vi "UI_Status.vi"(7 "write?":bool, 8 "error in (no error)":errorcluster caption="错误输入（无错误）", 10 "menu status in":T1={"type"=2, "scantime"=30, "highspd"=FALSE, "disp"=TRUE, "save"=FALSE, "hl"=FALSE, "ID合并"=FALSE, "Rfun"=2, "Tfun"=2, "chk1"=FALSE, "chk2"=FALSE, "format"=enum."hex", "rateR1"=TRUE, "rateR2"=TRUE, "rateT1"=TRUE, "rateT2"=TRUE, "RcvE1"=TRUE, "RcvE2"=TRUE, "TSFormat"=enum."原始值", "RcvLen"=48}, 11 "VI ref":refnum<vi>) -> (0 "error out":errorcluster caption="错误输出", 3 "menu status in out":T1={"type"=2, "scantime"=30, "highspd"=FALSE, "disp"=TRUE, "save"=FALSE, "hl"=FALSE, "ID合并"=FALSE, "Rfun"=2, "Tfun"=2, "chk1"=FALSE, "chk2"=FALSE, "format"=enum."hex", "rateR1"=TRUE, "rateR2"=TRUE, "rateT1"=TRUE, "rateT2"=TRUE, "RcvE1"=TRUE, "RcvE2"=TRUE, "TSFormat"=enum."原始值", "RcvLen"=48})   [LabVIEW 2011]
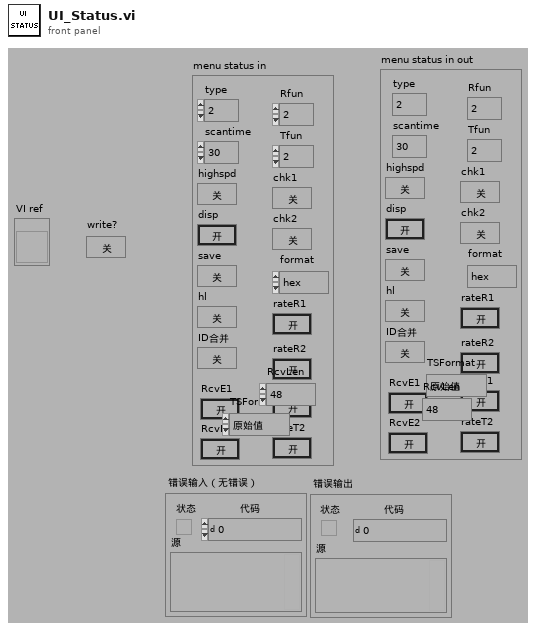
[diagram p1: front panel]
types:
  T1 = cluster{"type":u16, "scantime":u16, "highspd":bool, "disp":bool, "save":bool, "hl":bool, "ID合并":bool, "Rfun":u16, "Tfun":u16, "chk1":bool, "chk2":bool, "format":enum16{"hex", "dec", "oct", "bin"}, "rateR1":bool, "rateR2":bool, "rateT1":bool, "rateT2":bool, "RcvE1":bool, "RcvE2":bool, "TSFormat":enum16{"原始值", "实际值"}, "RcvLen":i16}
  T2 = cluster{"类ID":u32, "标签.文本":string, "禁用":enum8{"Enabled", "Disabled", "Disabled and Grayed Out"}, "可见":bool, "值":variant}[]
  T3 = cluster{"类ID":u32, "标签.文本":string, "禁用":enum8{"Enabled", "Disabled", "Disabled and Grayed Out"}, "可见":bool, "值":variant}
  T4 = enum8{"Enabled", "Disabled", "Disabled and Grayed Out"}
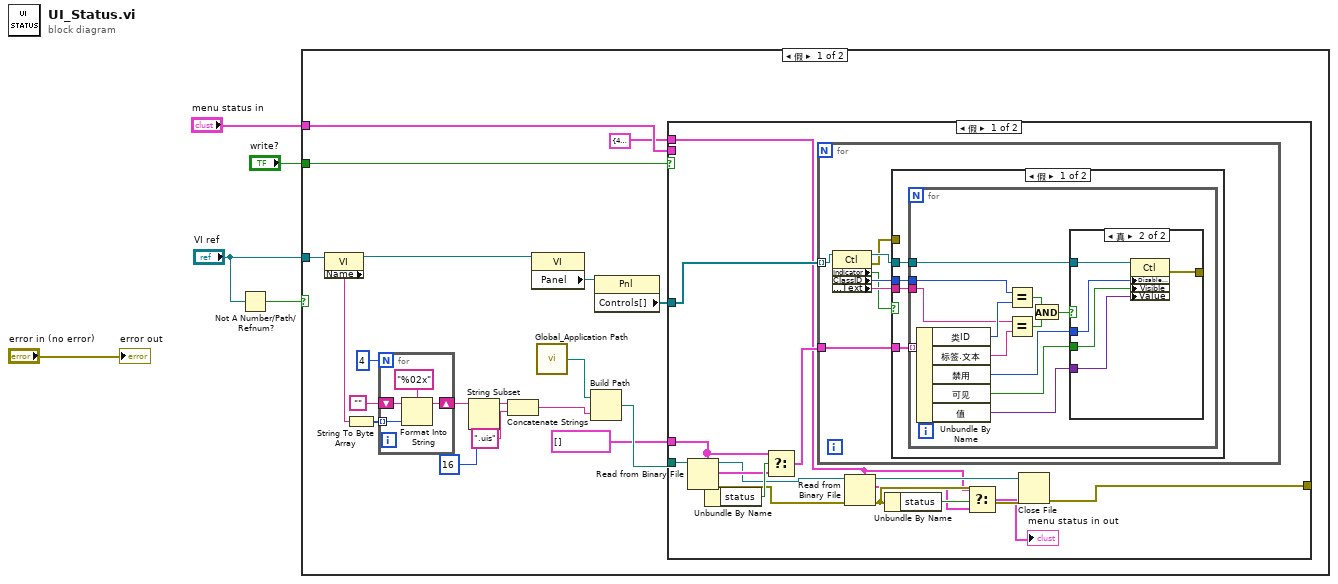
[diagram p0: block diagram]
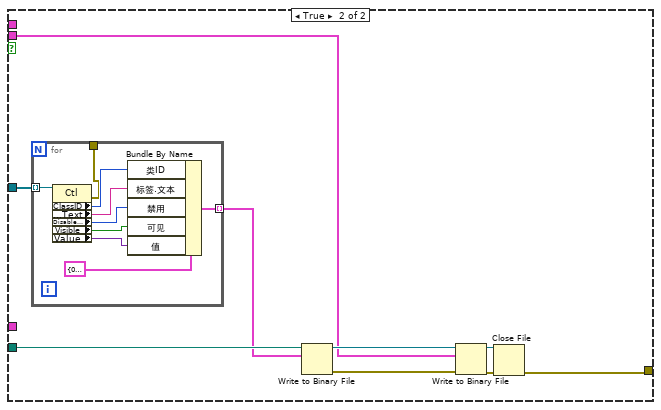
[diagram p4: hidden frame]
diagram:
  n1 = Not A Number/Path/Refnum?(number/path/refnum="VI ref") -> (NaN/Path/Refnum?=w1:bool)
  n2 = case shown="假" w1 {
    tunnel: "VI ref" -> [w24 _]
    tunnel: "write?" -> [w20 _]
    tunnel: "menu status in" -> [w17 _]
    frame False {
      n3 = property class="VI"(reference=w24) -> (reference out=w23:refnum<vi>, "Name"=w14:string)  [unwired: 1 in, 1 out]
      n4 = String To Byte Array(string=w14) -> (unsigned byte array=w15:u8[])
      n5 = for {
        N: 4 -> [_]
        tunnel: w15 -> [w28] mode=indexing
        shift-right: [w25] -> w13
        shift-left: "" -> [w26]
        n6 = Format Into String(format string="%02x" ("格式字符串"), initial string=w26, w28) -> (resulting string=w25:string)  [unwired: 1 in, 1 out]
      }
      n7 = String Subset(string=w13, length (rest)=16 ("长度（剩余）")) -> (substring=w10:string)  [unwired: 1 in]
      n8 = Concatenate Strings(w10, ".uis" ("字符串")) -> (w11:string)
      n9 = property class="VI"(reference=w23) -> ("Panel"=w22:refnum<vi>)  [unwired: 1 in, 2 out]
      n10 = call "Global_Application Path.vi"() -> ("程序路径"=w8:path)  [unwired: 1 in]
      n11 = Build Path(base path=w8, name or relative path=w11) -> (appended path=w19:path)
      n12 = property class="Pnl"(reference=w22) -> ("Controls[]"=w21:refnum<vi>[])  [unwired: 1 in, 2 out]
      n13 = case shown="假" w20 {
        tunnel: w21 -> [w37 w80]
        tunnel: w19 -> [w43 w79]
        tunnel: T2 [] -> [w41 _]
        tunnel: [w39 w77] -> _
        tunnel: T1 {"type"=4, "scantime"=30, "highspd"=FALSE, "disp"=TRUE, "save"=FALSE, "hl"=FALSE, "ID合并"=FALSE, "Rfun"=2, "Tfun"=2, "chk1"=FALSE, "chk2"=FALSE, "format"=enum."hex", "rateR1"=TRUE, "rateR2"=TRUE, "rateT1"=TRUE, "rateT2"=TRUE, "RcvE1"=TRUE, "RcvE2"=TRUE, "TSFormat"=enum."原始值", "RcvLen"=2500} ("menu status in out") -> [w31 _]
        tunnel: w17 -> [_ w72]
        frame False {
          n14 = Read from Binary File(5:w41, 11:w43) -> (0:w34:errorcluster, 2:w40:T2, 3:w36:refnum<file>)  [unwired: 4 in, 1 out]
          n15 = Unbundle By Name(w34) -> ("status"=w42:bool)
          n16 = Select(t=w41, s=w42, f=w40) -> (s? t:f=w38:T2)
          n17 = for {
            tunnel: w38 -> [w49]
            tunnel: w37 -> [w50] mode=indexing
            n18 = property class="Ctl"(reference=w50) -> (reference out=w48:refnum<vi>, error out=w44:errorcluster, "Indicator"=w45:bool, "ClassID"=w47:u32, "Label.Text"=w46:string)  [unwired: 1 in]
            n19 = case shown="假" w45 {
              tunnel: w49 -> [w54 _]
              tunnel: w48 -> [w53 _]
              tunnel: w47 -> [w52 _]
              tunnel: w46 -> [w51 _]
              tunnel: w44 -> [_ _]
              frame False {
                n20 = for {
                  tunnel: w54 -> [w66] mode=indexing
                  tunnel: w53 -> [w58]
                  tunnel: w52 -> [w65]
                  tunnel: w51 -> [w63]
                  n21 = Unbundle By Name(w66) -> ("类ID"=w64:u32, "标签.文本"=w62:string, "禁用"=w57:T4, "可见"=w56:bool, "值"=w55:variant)
                  n22 = Equal?(x=w65, y=w64) -> (x = y?=w61:bool)
                  n23 = Equal?(x=w63, y=w62) -> (x = y?=w60:bool)
                  n24 = And(x=w61, y=w60) -> (x .and. y?=w59:bool)
                  n25 = case shown="真" w59 {
                    tunnel: w58 -> [_ w71]
                    tunnel: w57 -> [_ w70]
                    tunnel: w56 -> [_ w69]
                    tunnel: w55 -> [_ w68]
                    tunnel: [_ w67] -> _
                    frame False {
                    }
                    frame True {
                      n26 = property class="Ctl"(reference=w71, "DisabledEnum"=w70, "Visible"=w69, "Value"=w68) -> (error out=w67:errorcluster)  [unwired: 1 in, 1 out]
                    }
                  }
                }
              }
              frame True {
              }
            }
          }
          n27 = Read from Binary File(5:w31, 8:w34, 11:w36) -> (0:w33:errorcluster, 2:w30:T1, 3:w35:refnum<file>)  [unwired: 3 in, 1 out]
          n28 = Unbundle By Name(w33) -> ("status"=w32:bool)
          n29 = Select(t=w31, s=w32, f=w30) -> (s? t:f=→"menu status in out":T1)
          n30 = Close File(refnum=w35, error in=w33) -> (error out=w39:errorcluster)  [unwired: 1 out]
        }
        frame True {
          n31 = for {
            tunnel: w80 -> [w89] mode=indexing
            tunnel: [w82] -> w78 mode=indexing
            tunnel: [w81] -> _
            n32 = property class="Ctl"(reference=w89) -> (error out=w81:errorcluster, "ClassID"=w83:u32, "Label.Text"=w84:string, "DisabledEnum"=w85:T4, "Visible"=w86:bool, "Value"=w87:variant)  [unwired: 1 in, 1 out]
            n33 = Bundle By Name(cluster=T3 {"类ID"=0, "标签.文本"="", "禁用"=enum."Enabled", "可见"=FALSE, "值"=variant}, "类ID"=w83, "标签.文本"=w84, "禁用"=w85, "可见"=w86, "值"=w87) -> (w82:T3)
          }
          n34 = Write to Binary File(file (use dialog)=w79, data=w78) -> (refnum out=w76:refnum<file>, error out=w75:errorcluster)  [unwired: 4 in, 1 out]
          n35 = Write to Binary File(file (use dialog)=w76, data=w72, error in=w75) -> (refnum out=w74:refnum<file>, error out=w73:errorcluster)  [unwired: 3 in, 1 out]
          n36 = Close File(refnum=w74, error in=w73) -> (error out=w77:errorcluster)  [unwired: 1 out]
        }
      }
    }
    frame True {
    }
  }
  "error out" <- "error in (no error)"
